vi "Restart Skywire Dev Kit Serial J14 USB COM30 Port no use.vi"(8 "error in (no error)":errorcluster, 11 "Device Hardware ID":string="*VID_0403*PID_6001*") -> (0 "error out":errorcluster, 3 "Command Output":string)   [LabVIEW 2013]
doc: "This VI can restart a usb device or disconnect first then scan for new device."
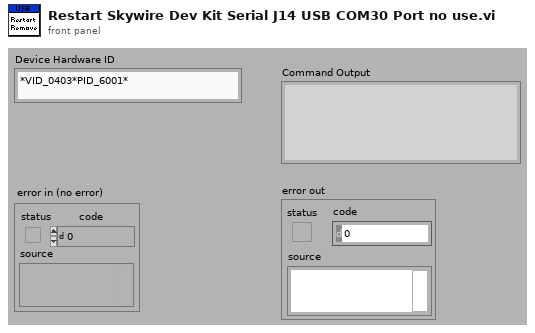
[diagram p1: front panel]
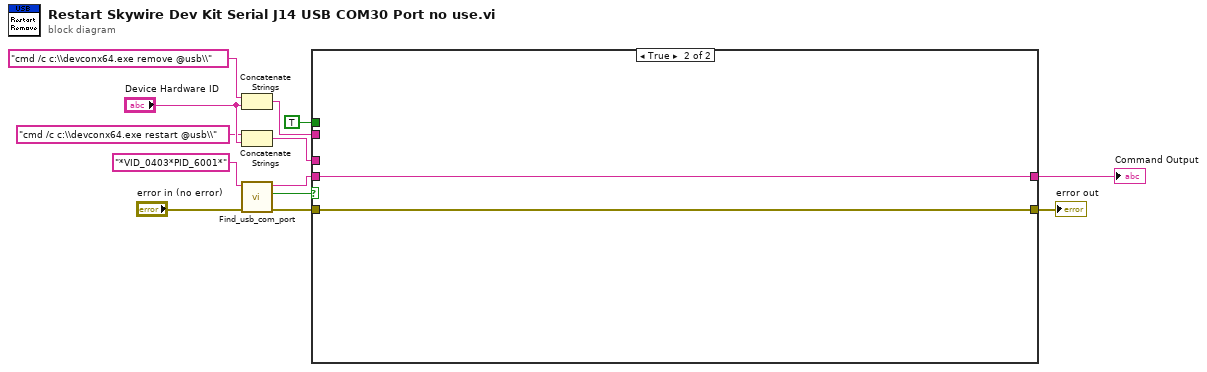
[diagram p0: block diagram]
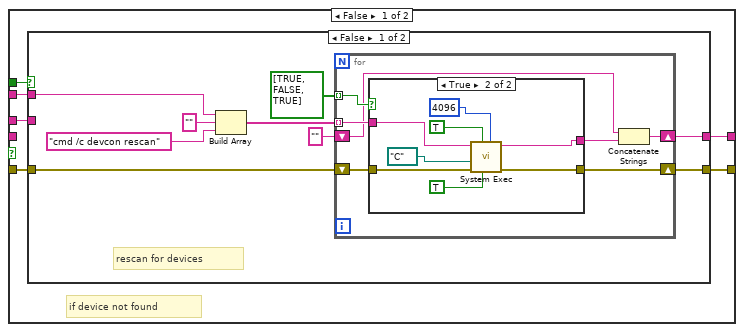
[diagram p2: hidden frame]
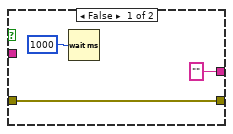
[diagram p3: hidden frame]
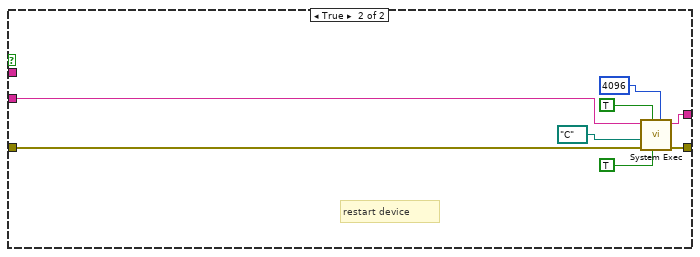
[diagram p4: hidden frame]
diagram:
  n1 = Concatenate Strings("cmd /c c:\\devconx64.exe remove @usb\\" ("command line"), "Device Hardware ID") -> (w12:string)
  n2 = Concatenate Strings("cmd /c c:\\devconx64.exe restart @usb\\" ("command line"), "Device Hardware ID") -> (w9:string)
  n3 = call "Find_usb_com_port.vi"("error in (no error)"="error in (no error)", "USB search key"="*VID_0403*PID_6001*" ("Device Hardware ID")) -> ("error out"=w3:errorcluster, "Found device"=w2:bool, "Comport"=w1:string)  [unwired: 7 in]
  n4 = case shown="True" w2 {
    tunnel: w12 -> [w19 _]
    tunnel: w9 -> [w18 _]
    tunnel: [w17 w55] -> w8
    tunnel: [w16 w56] -> w7
    tunnel: TRUE -> [w15 _]
    tunnel: w3 -> [w14 w56]
    tunnel: w1 -> [_ w55]
    frame False {
      # "if device not found"
      n5 = case shown="False" w15 {
        tunnel: w19 -> [w28 _]
        tunnel: w18 -> [_ w51]
        tunnel: [w21 w50] -> w16
        tunnel: w14 -> [w25 w49]
        tunnel: [w20 w48] -> w17
        frame False {
          # "rescan for devices"
          n6 = Build Array(w28, "", "cmd /c devcon rescan" ("command line")) -> (w24:string[])
          n7 = for {
            shift-right: [w35] -> w21
            shift-left: w25 -> [w34]
            tunnel: w24 -> [w33] mode=indexing
            tunnel: bool[] [TRUE, FALSE, TRUE] -> [w32] mode=indexing
            shift-right: [w29] -> w20
            shift-left: "" ("standard output") -> [w31]
            n8 = case shown="True" w32 {
              tunnel: ["" ("standard output") w45] -> w30
              tunnel: [w38 w44] -> w35
              tunnel: w34 -> [w38 w41]
              tunnel: w33 -> [_ w40]
              frame False {
                n9 = Wait (ms)(milliseconds to wait=u32 1000) -> ()  [unwired: 1 out]
              }
              frame True {
                n10 = call <vilib>:"System Exec.vi"("expected output size  (4096)"=u32 4096, "run minimized? (F)"=TRUE, "wait until completion? (T)"=TRUE, "error in (no error)"=w41, "working directory"=path "C:/", "command line"=w40) -> ("error out"=w44:errorcluster, "standard output"=w45:string)  [unwired: 2 in, 2 out]
              }
            }
            n11 = Concatenate Strings(w31, w30) -> (w29:string)
          }
        }
        frame True {
          # "restart device"
          n12 = call <vilib>:"System Exec.vi"("expected output size  (4096)"=u32 4096, "run minimized? (F)"=TRUE, "wait until completion? (T)"=TRUE, "error in (no error)"=w49, "working directory"=path "C:/", "command line"=w51) -> ("error out"=w50:errorcluster, "standard output"=w48:string)  [unwired: 2 in, 2 out]
        }
      }
    }
    frame True {
    }
  }
  "Command Output" <- w8
  "error out" <- w7
